vi "Open-Save Alias Definitions.vi"(6 "Open (F)/ Save":bool, 7 "Dialog? (F)":bool, 8 "Error In":errorcluster, 9 "Descriptions Array in":string[](array[string]), 10 "Definitions Array in":string[](array[string]), 11 "Aliases Array in":string[](array[string])) -> (0 "Error Out":errorcluster, 1 "Descriptions Array out":string[](array[string]), 2 "Definitions Array out":string[](array[string]), 3 "Aliases Array out":string[](array[string]), 5 "File Content":string[](array[string]))   [LabVIEW 2021, in "Formula.lvlib"]
uses:
  Formula.lvlib
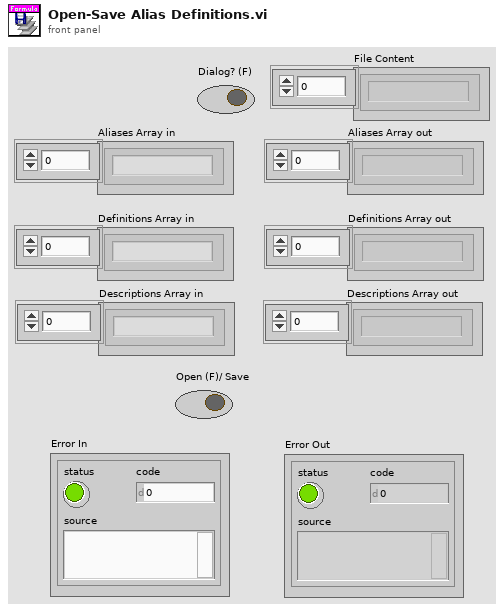
[diagram p1: front panel]
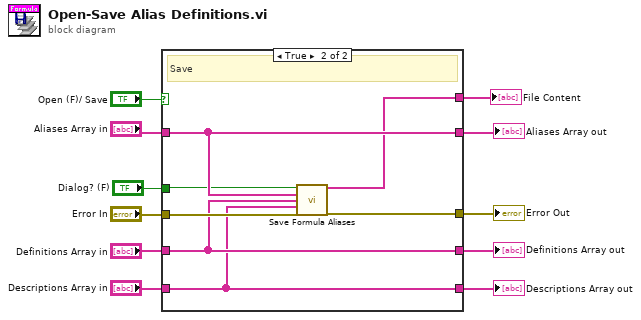
[diagram p0: block diagram]
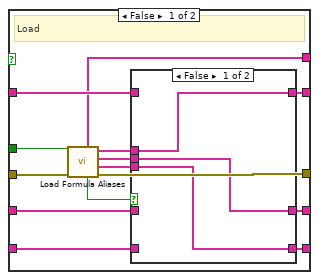
[diagram p2: hidden frame]
diagram:
  n1 = case shown="True" "Open (F)/ Save" {
    tunnel: "Error In" -> [w25 w38]
    tunnel: [w24 w35] -> w11
    tunnel: [w21 w37] -> w9
    tunnel: [w19 w36] -> w8
    tunnel: "Aliases Array in" -> [w22 w37]
    tunnel: "Definitions Array in" -> [w20 w36]
    tunnel: "Descriptions Array in" -> [w18 w34]
    tunnel: [w17 w34] -> w4
    tunnel: "Dialog? (F)" -> [w13 w33]
    tunnel: [w12 w32] -> w1
    frame False {
      # "Load"
      n2 = call "Load Formula Aliases.vi"("error in (no error)"=w25, "Dialog? (F)"=w13) -> ("error out"=w24:errorcluster, "Descriptions Array"=w14:string[], "Definitions Array"=w15:string[], "Aliases Array"=w16:string[], "Cancelled/Error"=w23:bool, "File Content"=w12:string[])  [unwired: 4 in]
      n3 = case shown="False" w23 {
        tunnel: w22 -> [_ w31]
        tunnel: [w28 w31] -> w21
        tunnel: w20 -> [_ w30]
        tunnel: [w27 w30] -> w19
        tunnel: w18 -> [_ w29]
        tunnel: [w26 w29] -> w17
        tunnel: w16 -> [w28 _]
        tunnel: w15 -> [w27 _]
        tunnel: w14 -> [w26 _]
        frame False {
        }
        frame True {
        }
      }
    }
    frame True {
      # "Save"
      n4 = call "Save Formula Aliases.vi"("Dialog? (F)"=w33, "Aliases Array"=w37, "Definitions Array"=w36, "Descriptions Array"=w34, "error in (no error)"=w38) -> ("File Content"=w32:string[], "error out"=w35:errorcluster)  [unwired: 9 in]
    }
  }
  "Definitions Array out" <- w8
  "Aliases Array out" <- w9
  "Error Out" <- w11
  "Descriptions Array out" <- w4
  "File Content" <- w1
